vi "Data Storage Through Reference.vi"(9 "Time Out In ms":i32=-1, 10 "Data In":T1, 11 "DVR In":refnum<data-value>) -> (1 "Time Out":bool, 3 "DVR Out":refnum<data-value>)   [LabVIEW 2019, in "2D U16 Group With ID DVR Queue.lvclass"]
uses:
  2D U16 Group With ID DVR Queue.lvclass
  Type Def/Data Type.ctl
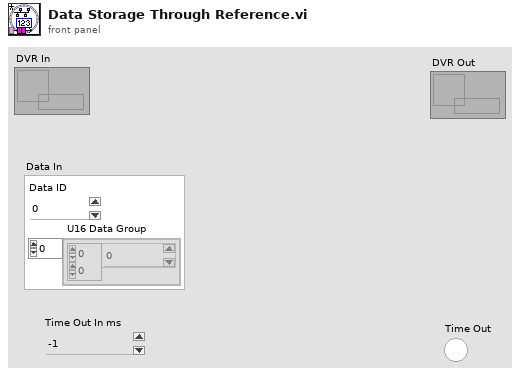
[diagram p1: front panel]
types:
  T1 = typedef "Data Type.ctl" = cluster{"Data ID":i64, "U16 Data Group":cluster{"Array":u16[][]}[]}
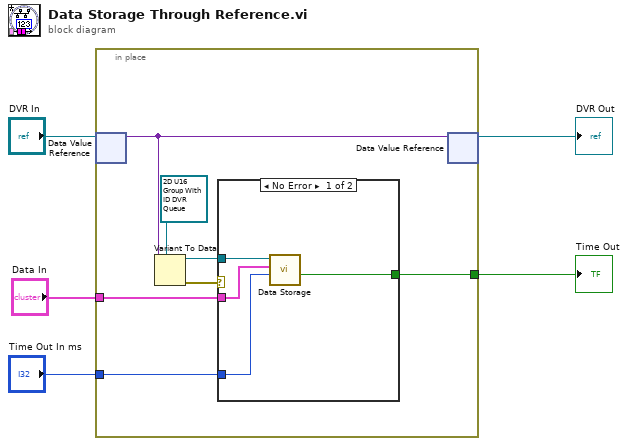
[diagram p0: block diagram]
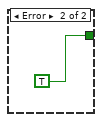
[diagram p2: hidden frame]
diagram:
  n1 = in-place {
    in-place-border: "Time Out In ms" -> [w9]
    in-place-border: [w8] -> w2
    in-place-border: "Data In" -> [w6]
    n2 = in-place-dvr #1("DVR In") -> (w12:variant)  [unwired: 1 out]
    n3 = Variant To Data(type=refnum<class "2D U16 Group With ID DVR Queue.lvclass"> refnum ("1D U16 Group With ID DVR Queue.lvclass"), Variant=w12) -> (data=w10:refnum<class "2D U16 Group With ID DVR Queue.lvclass">, error out=w11:errorcluster)  [unwired: 1 in]
    n4 = case shown="No Error" w11 {
      tunnel: w10 -> [w16 _]
      tunnel: w9 -> [w14 _]
      tunnel: [w15 TRUE ("Time Out")] -> w8
      tunnel: w6 -> [w13 _]
      frame No Error {
        n5 = call "Data Storage.vi"("Time Out In ms"=w14, "Data In"=w13, "1D U16 Group With ID DVR Queue in"=w16) -> ("Time Out"=w15:bool)  [unwired: 7 in, 1 out]
      }
      frame Error {
      }
    }
    n6 = in-place-dvr #1(w12) -> (→"DVR Out":refnum<data-value>)  [unwired: 1 out]
  }
  "Time Out" <- w2
